vi "PH_BL-Master.Set Ready to Shot.vi"(0 "i ref in":refnum<vi>, 2 "R2S?":bool, 5 "error in (no error)":errorcluster) -> (14 "i ref out":refnum<vi>, 19 "error out":errorcluster)   [LabVIEW 2014, in "PH_BL-Master.lvlib"]
doc: "This VI sets whether the R2S-Information (\"ready to shot\") to own attributes, and publishes it as DIM service."
uses:
  PH_BL-Master.lvlib
  PH_Common/PH_Common.lvlib
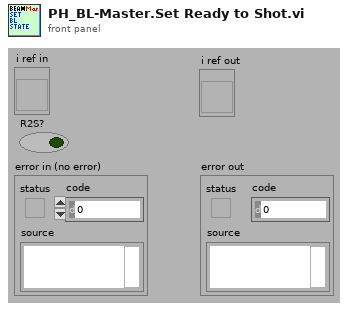
[diagram p1: front panel]
types:
  T1 = typedef "PH_BL-Master.lvlib/PH_BL-Master.i attribute.ctl" = cluster{"Remote controlled":bool, "Boolean Condition Service Subscriber":refnum<vi>[], "Picture Condition Service Subscriber":refnum<vi>[], "R2S":cluster{"GUI Ref":refnum<vi>, "State":bool}, "Vacua":cluster{"GUI Ref":refnum<vi>, "Limit":dbl, "Curr Value":dbl, "in range":bool}[], "O2 Inspection":cluster{"GUI Ref":refnum<vi>, "Concentration":dbl, "State":T2}[], "Boolean Status Service Subscriber":cluster{"GUI Ref":refnum<vi>, "Status":T2, "no Link?":bool, "Status Subscriber Class":T3}[], "Picture Status Service Subscriber":cluster{"GUI Ref":refnum<vi>, "Status":T2, "no Link?":bool, "Status Subscriber Class":T3}[], "6P 4Q Service Subscriber":cluster{"GUI Ref":refnum<vi>, "Selector":T4, "no Link?":bool}[], "Index of latest 6P 4Q changing Instance":i32, "Index of latest Picture Status changing Instance":i32, "Index of latest Boolean Status changing Instance":i32, "Vision ID on same Node":string, "Start Phase over?":bool, "GUI Ref Delete":refnum<vi>}
  T2 = typedef "PH_StatusHandler.lvlib/PH_StatusHandler.Status.ctl" = i16
  T3 = typedef "PH_BL-Master.lvlib/PH_BL-Master.Status Subscriber Class.ctl" = enum16{"unknown", "Switch", "BB", "6P Switch", "Switch GUI", "Switch and 6P State", "Force Sensor"}
  T4 = typedef "PH_4_Pos_Selector.lvlib/PH_4_Pos_Selector.Position Selector.ctl" = u16
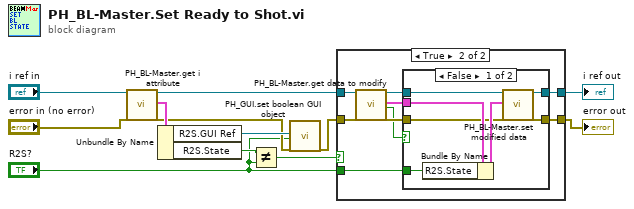
[diagram p0: block diagram]
diagram:
  n1 = call "PH_BL-Master.get i attribute.vi"("i ref in"="i ref in", "error in (no error)"="error in (no error)") -> ("i ref out"=w7:refnum<vi>, "i attribute"=w10:T1, "error out"=w4:errorcluster)  [unwired: 15 in]
  n2 = Unbundle By Name(w10) -> ("R2S.GUI Ref"=w5:refnum<vi>, "R2S.State"=w2:bool)
  n3 = Not Equal?(x=w2, y="R2S?") -> (x != y?=w6:bool)
  n4 = call "PH_GUI.set boolean GUI object.vi"("Boolean Knob GUI Ref"=w5, "Value"="R2S?", "error in (no error)"=w4) -> ("error out"=w3:errorcluster)  [unwired: 16 in]
  n5 = case shown="True" w6 {
    tunnel: [w14 w21] -> w12
    tunnel: [w13 w20] -> w11
    tunnel: w3 -> [w13 w17]
    tunnel: w7 -> [w14 w16]
    tunnel: "R2S?" -> [_ w15]
    frame False {
    }
    frame True {
      n6 = call "PH_BL-Master.get data to modify.vi"("i ref in"=w16, "error in (no error)"=w17) -> ("i ref out"=w22:refnum<vi>, "i attribute"=w19:T1, "timed out"=w18:bool, "error out"=w23:errorcluster)  [unwired: 14 in]
      n7 = case shown="False" w18 {
        tunnel: w23 -> [w24 w31]
        tunnel: w22 -> [w30 w32]
        tunnel: [w29 w32] -> w21
        tunnel: [w28 w31] -> w20
        tunnel: w19 -> [w27 _]
        tunnel: w15 -> [w25 _]
        frame False {
          n8 = Bundle By Name(cluster=w27, "R2S.State"=w25) -> (w26:T1)
          n9 = call "PH_BL-Master.set modified data.vi"("i ref in"=w30, "i attribute"=w26, "error in (no error)"=w24) -> ("i ref out"=w29:refnum<vi>, "error out"=w28:errorcluster)  [unwired: 15 in]
        }
        frame True {
        }
      }
    }
  }
  "error out" <- w11
  "i ref out" <- w12
